vi "end_point_calculation.vi"(8 "bucket":dbl, 9 "arm":dbl, 10 "boom":dbl) -> ()   [LabVIEW 2020]
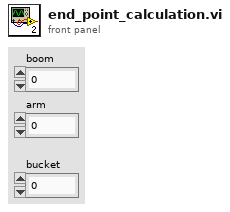
[diagram p1: front panel]
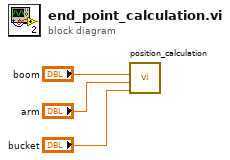
[diagram p0: block diagram]
diagram:
  n1 = call "position_calculation.vi"("bucket_angle"="bucket", "arm_angle"="arm", "boom_angle"="boom") -> ()  [unwired: 8 in, 1 out]
